vi "FP RT main.vi"() -> ()   [LabVIEW 2014]
uses:
  <vilib>/userdefined/High Color/IMAQdx.ctl
  <vilib>/myRIO/Instrument Drivers/Onboard IO/PWM/typedefs/PWM Reference.ctl
  <vilib>/myRIO/Common/Instrument Driver Framework/Utilities/typedefs/myRIO Generic Hardware Reference.ctl
  <vilib>/myRIO/Common/Instrument Driver Framework/Utilities/typedefs/Hardware Version Enum.ctl
  <vilib>/myRIO/Common/Instrument Driver Framework/Utilities/typedefs/myRIO v1.0 Reference.ctl
  <vilib>/myRIO/Common/Instrument Driver Framework/Utilities/typedefs/Generic FPGA Reference.ctl
  <vilib>/myRIO/Common/Instrument Driver Framework/myRIO v1.0/PWM/typedefs/PWM Channels Enum.ctl
  <vilib>/myRIO/Instrument Drivers/Onboard IO/PWM/typedefs/PWM Configuration.ctl
  <vilib>/userdefined/High Color/nirio_resource_hc.ctl
  <vilib>/myRIO/Instrument Drivers/Onboard IO/DIO/typedefs/DIO Reference.ctl
  <vilib>/myRIO/Common/Instrument Driver Framework/myRIO v1.0/DIO/typedefs/DIO Channels List.ctl
  <vilib>/myRIO/Common/Instrument Driver Framework/myRIO v1.0/DIO/typedefs/DIO Channels Enum.ctl
  <vilib>/myRIO/Instrument Drivers/Onboard IO/AI/typedefs/AI Reference.ctl
  <vilib>/myRIO/Common/Instrument Driver Framework/myRIO v1.0/AI/typedefs/AI Channels List.ctl
  <vilib>/myRIO/Common/Instrument Driver Framework/myRIO v1.0/AI/typedefs/AI Channels Enum.ctl
  <vilib>/myRIO/Common/Instrument Driver Framework/Utilities/typedefs/Analog Scaling Constants List.ctl
  <vilib>/myRIO/Common/Instrument Driver Framework/Utilities/typedefs/Analog Scaling Constants.ctl
  <vilib>/myRIO/Common/Instrument Driver Framework/myRIO v1.0/PWM/vis/myRIO v1.1 Open PWM.vi
  <vilib>/myRIO/Common/Instrument Driver Framework/myRIO v1.0/DIO/vis/myRIO v1.1 Open DIO.vi
  <vilib>/myRIO/Common/Instrument Driver Framework/myRIO v1.0/AI/vis/myRIO v1.1 Open AI.vi
  <vilib>/myRIO/Common/Instrument Driver Framework/Utilities/vis/Validate Channels.vi
  <vilib>/myRIO/Common/Instrument Driver Framework/myRIO v1.0/PWM/vis/myRIO v1.0 Reserve PWM.vi
  <vilib>/myRIO/Common/Instrument Driver Framework/myRIO v1.0/DIO/vis/myRIO v1.0 Reserve DIO.vi
  <vilib>/myRIO/Common/Instrument Driver Framework/myRIO v1.0/AI/vis/myRIO v1.0 Reserve AI.vi
  <vilib>/myRIO/Common/Instrument Driver Framework/myRIO v1.0/PWM/vis/myRIO v1.0 Close PWM.vi
  <vilib>/myRIO/Common/Instrument Driver Framework/myRIO v1.0/DIO/vis/myRIO v1.0 Close DIO.vi
  <vilib>/myRIO/Common/Instrument Driver Framework/myRIO v1.0/AI/vis/myRIO v1.0 Close AI.vi
  <vilib>/myRIO/Common/Instrument Driver Framework/myRIO v1.0/PWM/vis/myRIO v1.0 Build MUX Configuration PWM.vi
  <vilib>/myRIO/Common/Instrument Driver Framework/myRIO v1.0/Resource Manager/vis/myRIO v1.0 Reserve Channel List.vi
  <vilib>/myRIO/Common/Instrument Driver Framework/myRIO v1.0/DIO/vis/myRIO v1.0 Build MUX Configuration DIO.vi
  <vilib>/myRIO/Common/Instrument Driver Framework/myRIO v1.0/AI/vis/myRIO v1.0 Build MUX Configuration AI.vi
  <vilib>/myRIO/Common/Instrument Driver Framework/myRIO v1.0/PWM/vis/myRIO v1.0 Unreserve PWM.vi
  <vilib>/myRIO/Common/Instrument Driver Framework/myRIO v1.0/DIO/vis/myRIO v1.0 Unreserve DIO.vi
  <vilib>/myRIO/Common/Instrument Driver Framework/myRIO v1.0/AI/vis/myRIO v1.0 Unreserve AI.vi
  <vilib>/myRIO/Common/Instrument Driver Framework/myRIO v1.0/Resource Manager/vis/myRIO v1.0 Create Configuration List.vi
  <vilib>/myRIO/Common/Instrument Driver Framework/myRIO v1.0/Resource Manager/vis/myRIO v1.0 Reserve Channel.vi
  <vilib>/myRIO/Common/Instrument Driver Framework/myRIO v1.0/Resource Manager/vis/myRIO v1.0 Unreserve Channel.vi
  <vilib>/myRIO/Common/Instrument Driver Framework/myRIO v1.0/Resource Manager/vis/myRIO v1.0 Unreserve Channel List.vi
  <vilib>/myRIO/Common/Instrument Driver Framework/myRIO v1.0/Resource Manager/vis/myRIO v1.0 Build Mutex Name.vi
  <vilib>/Utility/VariantDataType/GetNumericInfo.vi
  <vilib>/Utility/error.llb/Error Cluster From Error Code.vi
  <vilib>/myRIO/Common/Instrument Driver Framework/myRIO v1.0/myRIO v1.1 Open.vi
  <vilib>/myRIO/Common/Instrument Driver Framework/myRIO v1.0/AI/vis/myRIO v1.0 Get Scaling Constants AI.vi
  <vilib>/myRIO/Common/Instrument Driver Framework/Utilities/vis/IO Manager.vi
  <vilib>/myRIO/Common/Instrument Driver Framework/Utilities/vis/Configuration Manager.vi
  <vilib>/myRIO/Common/Instrument Driver Framework/myRIO v1.0/myRIO v1.0 Close.vi
  <vilib>/myRIO/Common/Instrument Driver Framework/myRIO v1.0/Resource Manager/vis/myRIO v1.0 Configure IO.vi
  <vilib>/myRIO/Common/Instrument Driver Framework/myRIO v1.0/AI/vis/myRIO v1.0 Read AI.vi
  <vilib>/myRIO/Common/Instrument Driver Framework/myRIO v1.0/DIO/vis/myRIO v1.0 Write DIO.vi
  <vilib>/myRIO/Common/Instrument Driver Framework/myRIO v1.0/PWM/vis/myRIO v1.0 Write PWM.vi
  <vilib>/myRIO/Common/Instrument Driver Framework/myRIO v1.0/PWM/vis/myRIO v1.0 Shutdown PWM.vi
  <vilib>/myRIO/Common/Instrument Driver Framework/myRIO v1.0/DIO/vis/myRIO v1.0 Shutdown DIO.vi
  <vilib>/myRIO/Instrument Drivers/Onboard IO/AI/vis/myRIO AI Open.xnode
  <vilib>/myRIO/Instrument Drivers/Onboard IO/DIO/vis/myRIO DIO Open.xnode
  <vilib>/myRIO/Instrument Drivers/Onboard IO/PWM/vis/myRIO PWM Open.xnode
  <vilib>/vision/driver/NI_Vision_Acquisition_Software.lvlib
  <vilib>/myRIO/Instrument Drivers/Onboard IO/AI/AI.lvlib
  <vilib>/myRIO/Instrument Drivers/Onboard IO/DIO/DIO.lvlib
  <vilib>/myRIO/Instrument Drivers/Onboard IO/PWM/PWM.lvlib
panel:
  in  "Waypoint seed":T1={"Type"=enum."Start", "X"=250, "Y"=250, "Speed"=0, "Behaviors"=enum."Open Water Transit"}
  in  "spyder":cluster{"magnitude":dbl, "phase":dbl}[](array[cluster]) {"phase" format="%0.2f"; "magnitude" format="%0.2f"}
  in  "Tab Control":T2(tab)
  out "GLED":bool
  out "BLED":bool
  out "RLED":bool
  out "BW Image":T3(plugin-control)
  in  "stop":bool
  out "Midbrain?":bool
  out "Rudder":dbl(knob) min=-45.0 max=45.0 step=1.0 scale=-45.0..45.0
  out "Speed":dbl(knob) min=-9.0 max=9.0 step=1.0 scale=-50.0..50.0
  out "Hindbrain?":bool
  out "Forebrain?":bool
  out "Battery Dead?":bool
  out "Complete?":bool=TRUE
  out "Arbiter Graph":cluster{dbl, dbl, dbl[]}(graph)
  in  "Session In":T4="cam0"
  out "Color Image":T3(plugin-control)
  out "Nb Circles":i32
  out "UDP Time Out?":bool
  in  "Tug letter":string="T"
  in  "Run?":bool
  in  "MSpeed":dbl(slide) scale=-50.0..50.0 scale format="%#.1g"
  in  "MHeading":dbl(slide) scale=-45.0..45.0 scale format="%_1f"
  in  "Manual?":bool
  out "Boat Status":T5={"GPS"={"X pos"=0, "Y pos"=0, "Heading"=0.0}, "IR Sensors"=[{"Name"="Bow", "Angle"=0.0, "Distance"=0.0}], "MOT BAT"=7.2, "RIO BAT"=7.2}
  out "GPS?":bool
  out "Camera Data":T6
  out "TA GPS":cluster{"X pos":i32, "Y pos":i32, "Heading":dbl}
  in  "TA Tug Letter":string="L"
  out "TAGPS?":bool
  out "Act Com":T7
  out "Forebrain ACT":dbl[](array[numeric])
  out "IR Sensors":T8(array[cluster])
  out "GPS":cluster{"X pos":i32, "Y pos":i32, "Heading":dbl}
  out "RED LED":bool
  out "GREEN LED":bool
  out "BLUE LED":bool
  in  "MDF":T9(array[cluster])=[{"Type"=enum."Start", "X"=250, "Y"=250, "Speed"=0, "Behaviors"=enum."Open Water Transit"}, {"Type"=enum."Waypoint", "X"=400, "Y"=100, "Speed"=20, "Behaviors"=enum."P-Wall Follow"}, {"Type"=enum."Waypoint", "X"=250, "Y"=250, "Speed"=20, "Behaviors"=enum."Open Water Transit"}, {"Type"=enum."Waypoint", "X"=250, "Y"=400, "Speed"=20, "Behaviors"=enum."Open Water Transit"}, {"Type"=enum."Waypoint", "X"=100, "Y"=400, "Speed"=20, "Behaviors"=enum."Open Water Transit"}, {"Type"=enum."End", "X"=250, "Y"=250, "Speed"=0, "Behaviors"=enum."Open Water Transit"}]
  out "GPS Initial":cluster{"X pos":i32, "Y pos":i32, "Heading":dbl}
  out "In chase mode?":bool
  out "Polar Plot":picture
  out "Invalid Pos?":bool
  out "error out":errorcluster
  out "Forebrain Comd":T10
  out "Debug IR \nRaw \nReadings":T8(array[cluster])
  out "Boat Speed":dbl format="%#_15g"
  in  "BOATPOS":T11
  in  "Boxcars":T12
  out "Chase MDF":T9(array[cluster])
  out "MDF INDEX CHASE":i32
  out "Docking MDF":T9(array[cluster])
  out "MDF INDEX DOCKING":i32
  out "MDF Active":T9(array[cluster])
  out "MDF INDEX":i32
  # "To start the Tug, press the \">\" key in the tool bar.\n\nPress the Run? control to start the Mission.\n\nWhen complete the Complete? indicator will light.\n\nIf the Run? is not pressed again, the mission will start again.\n\nAlways press the STOP button to end the operation!!!!!!!!!!!!!"
  # "Press the Manual? button to control\nthe Tug from the sliders"
  # "Stuck indicates that\nthe boat is not moving."
  # "Enter the Letter\nof  your Tug"
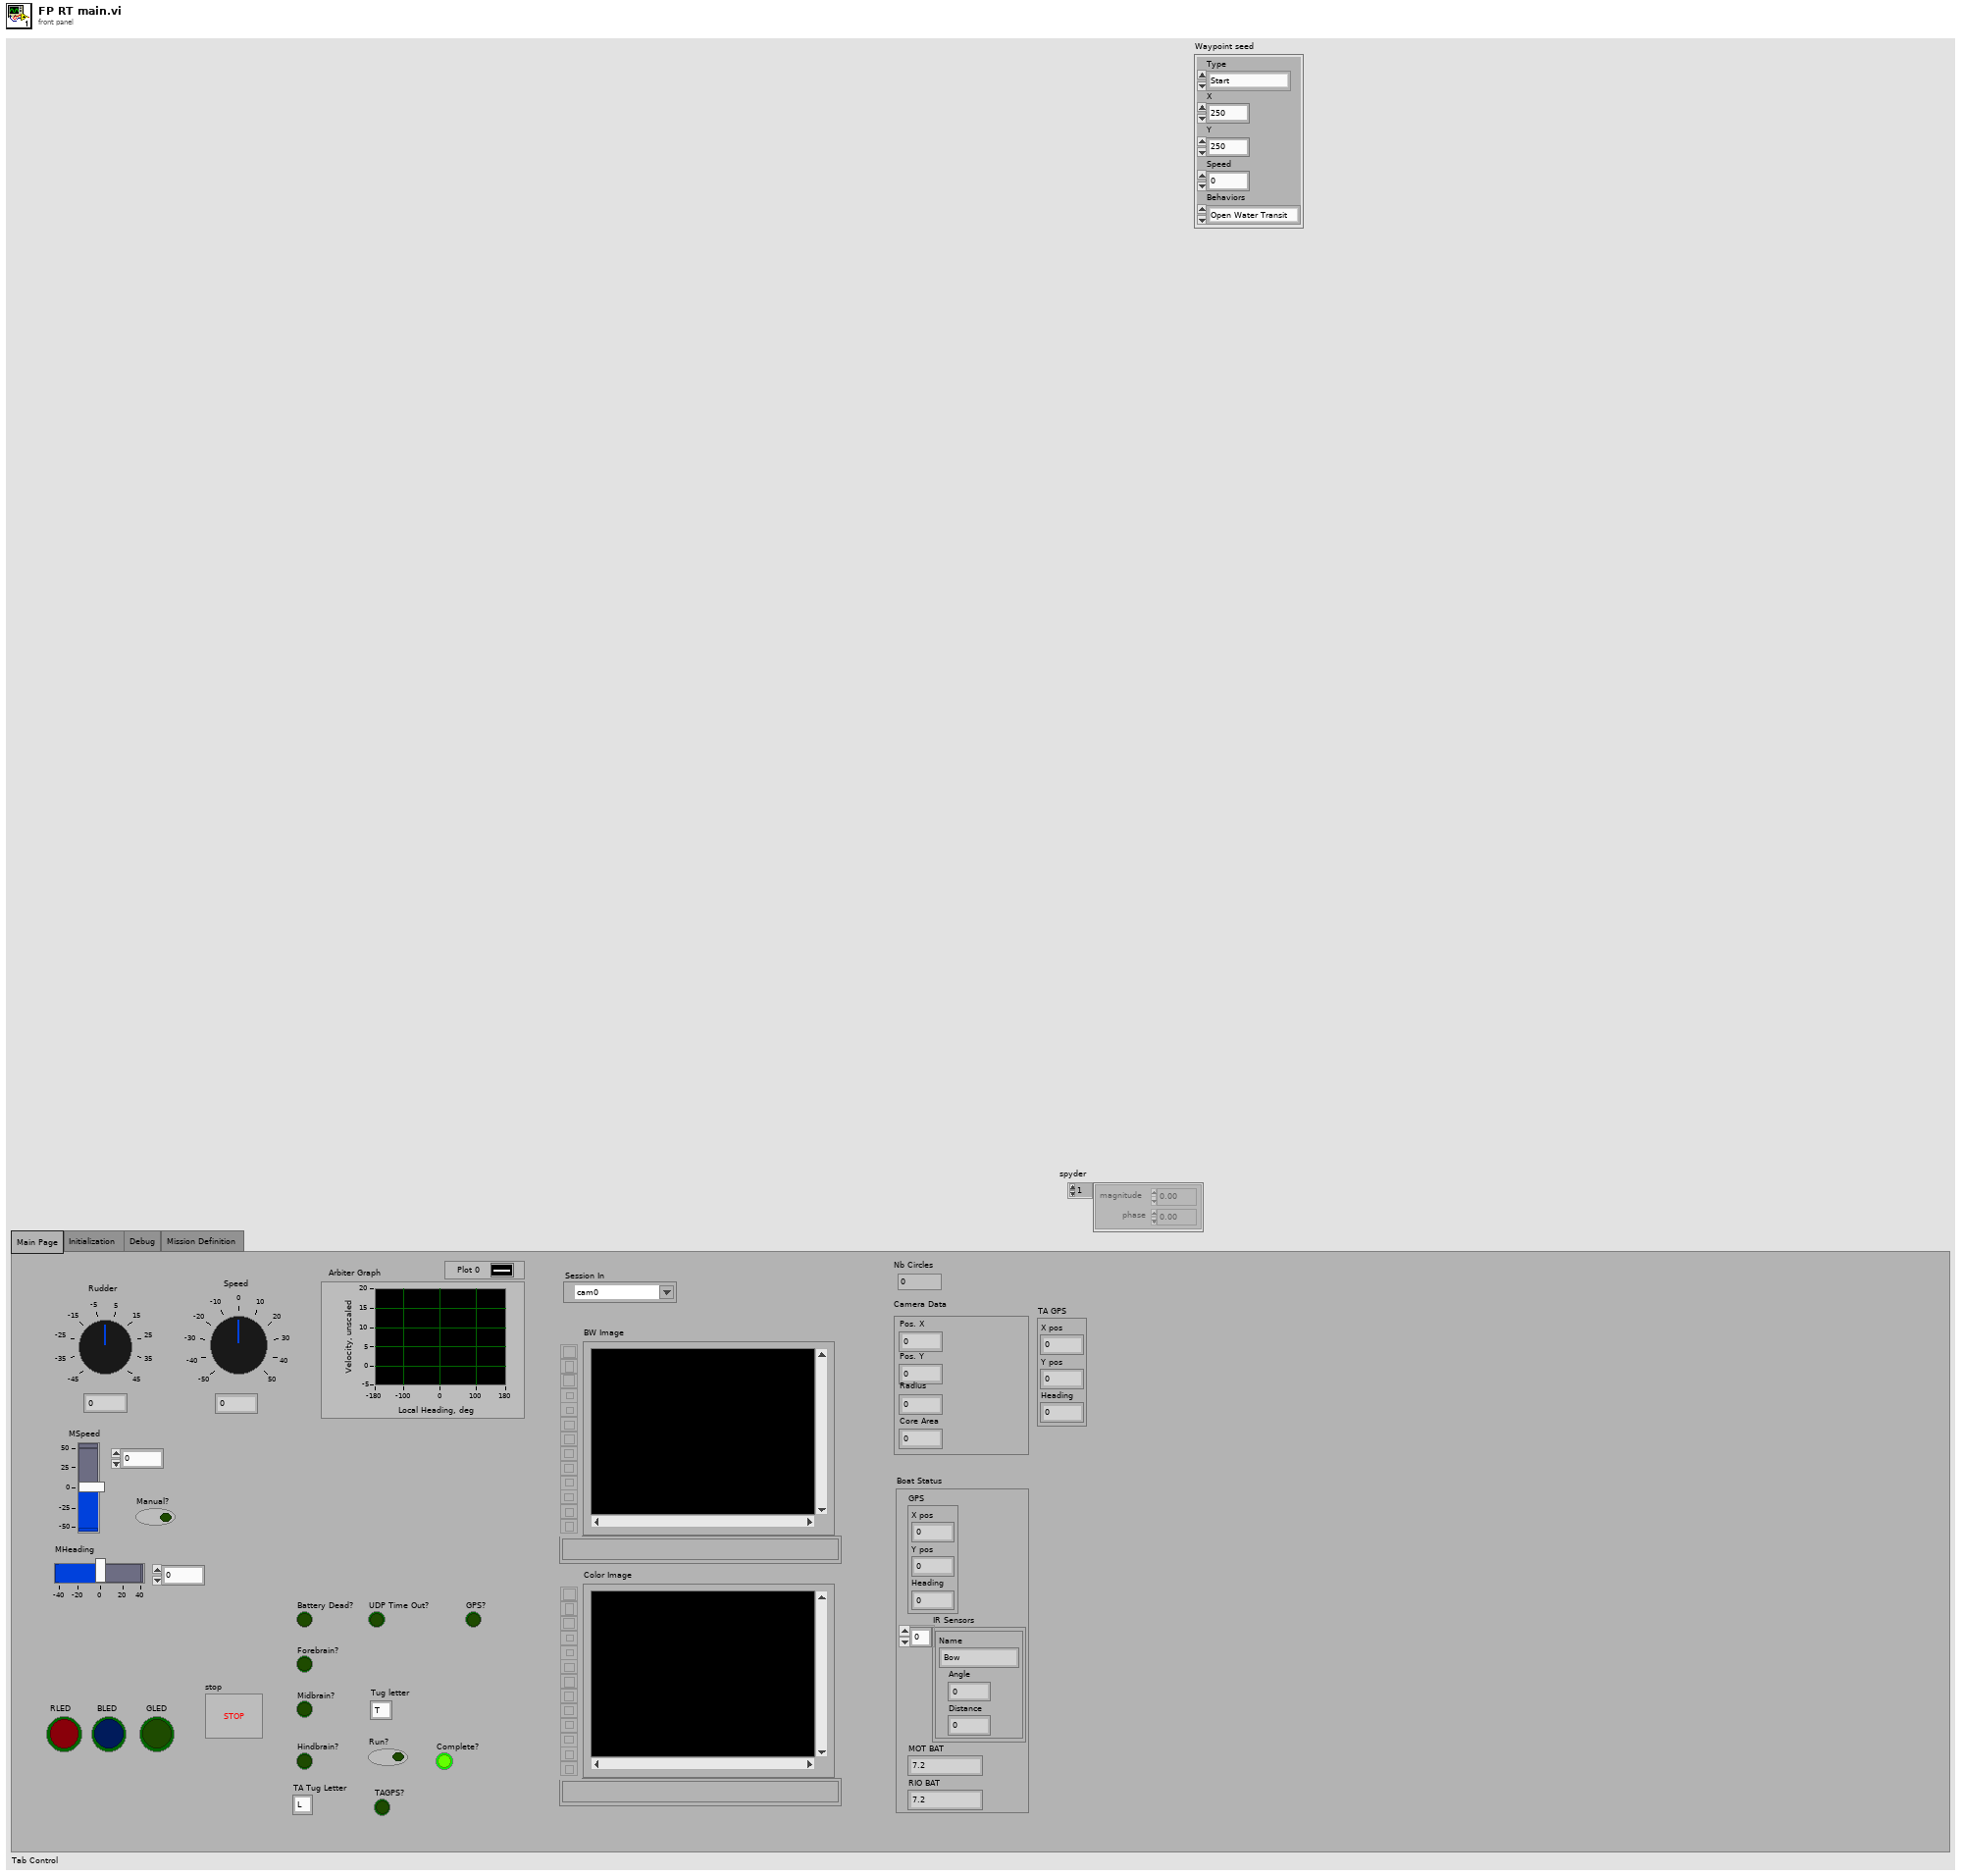
[diagram p1: front panel]
types:
  T1 = cluster{"Type":enum16{"Start", "Waypoint", "End"}, "X":i32, "Y":i32, "Speed":i32, "Behaviors":enum16{"Open Water Transit", "P-Wall Follow", "S-Wall Follow", "Dock", "Chase"}}
  T2 = enum32{"Main Page", "Initialization", "Debug", "Mission Definition"}
  T3 = typedef "IMAQ Image.ctl" = refnum<image>
  T4 = typedef "IMAQdx.ctl" = refnum<k21>
  T5 = cluster{"GPS":cluster{"X pos":i32, "Y pos":i32, "Heading":dbl}, "IR Sensors":cluster{"Name":string, "Angle":dbl, "Distance":dbl}[], "MOT BAT":dbl, "RIO BAT":dbl}
  T6 = cluster{"Pos. X":i32, "Pos. Y":i32, "Radius":i32, "Core Area":i32}
  T7 = cluster{"Desired Local\nHeading":dbl, "Desired\nSpeed":dbl}
  T8 = cluster{"Name":string, "Angle":dbl, "Distance":dbl}[]
  T9 = cluster{"Type":enum16{"Start", "Waypoint", "End"}, "X":i32, "Y":i32, "Speed":i32, "Behaviors":enum16{"Open Water Transit", "P-Wall Follow", "S-Wall Follow", "Dock", "Chase"}}[]
  T10 = cluster{"Behaviors":enum16{"Open Water Transit", "P-Wall Follow", "S-Wall Follow", "Dock", "Chase"}, "Behavior\nVelocity":dbl}
  T11 = cluster{"Old X Position":i32, "Old Y Position":i32}
  T12 = cluster{"IR Sensor Boxcars":dbl[][], "Boat Speed  Boxcars":dbl[]}
  T13 = cluster{"Type":enum16{"Start", "Waypoint", "End"}, "X":i32, "Y":i32, "Speed":i32, "Behaviors":enum16{"Open Water Transit", "P-Wall Follow", "S-Wall Follow", "Dock"}}[]
  T14 = typedef "nirio_resource_hc.ctl" = tag
  T15 = typedef "Hardware Version Enum.ctl" = enum16{"Unknown", "myRIO-1900", "myRIO-1950"}
  T16 = typedef "Image Type" = u32
  T17 = enum16{"Open Water Transit", "P-Wall Follow", "S-Wall Follow", "Dock", "Chase"}
  T18 = typedef "PWM.lvlib/PWM Reference.ctl" = cluster{"myRIO Reference":T19, "PWM Channels Enum":T22, "PWM Configuration":T23}
  T19 = typedef "myRIO Generic Hardware Reference.ctl" = cluster{"myRIO Model":T15, "myRIO Hardware Reference":T20}
  T20 = typedef "myRIO v1.0 Reference.ctl" = cluster{"Generic FPGA Reference":T21, "Allow multiple opens":bool}
  T21 = typedef "Generic FPGA Reference.ctl" = refnum<k20>
  T22 = typedef "PWM Channels Enum.ctl" = enum16{"Not Connected", "C/PWM0", "C/PWM1", "A/PWM0", "A/PWM1", "A/PWM2", "B/PWM0", "B/PWM1", "B/PWM2"}
  T23 = typedef "PWM.lvlib/PWM Configuration.ctl" = cluster{"Frequency":dbl, "Duty Cycle":dbl}
  T24 = typedef "DIO.lvlib/DIO Reference.ctl" = cluster{"myRIO Reference":T19, "DIO Channels List":T25}
  T25 = typedef "DIO Channels List.ctl" = T26[]
  T26 = typedef "DIO Channels Enum.ctl" = enum16{"Not Connected", "C/DIO0", "C/DIO1", "C/DIO2", "C/DIO3", "C/DIO4", "C/DIO5", "C/DIO6", "C/DIO7", "A/DIO0", "A/DIO1", "A/DIO2", "A/DIO3", "A/DIO4", "A/DIO5", "A/DIO6", "A/DIO7", "A/DIO8", "A/DIO9", "A/DIO10", "A/DIO11", "A/DIO12", "A/DIO13", "A/DIO14", "A/DIO15", "B/DIO0", "B/DIO1", "B/DIO2", "B/DIO3", "B/DIO4", "B/DIO5", "B/DIO6", "B/DIO7", "B/DIO8", "B/DIO9", "B/DIO10", "B/DIO11", "B/DIO12", "B/DIO13", "B/DIO14", "B/DIO15", "LED0", "LED1", "LED2", "LED3", "Button0"}
  T27 = typedef "AI.lvlib/AI Reference.ctl" = cluster{"myRIO Reference":T19, "AI Channels List":T28, "AI Scaling Constants List":T30}
  T28 = typedef "AI Channels List.ctl" = T29[]
  T29 = typedef "AI Channels Enum.ctl" = enum16{"Not Connected", "AudioIn/Left", "AudioIn/Right", "C/AI0", "C/AI1", "A/AI0", "A/AI1", "A/AI2", "A/AI3", "B/AI0", "B/AI1", "B/AI2", "B/AI3"}
  T30 = typedef "Analog Scaling Constants List.ctl" = T31[]
  T31 = typedef "Analog Scaling Constants.ctl" = cluster{"LSB Weight (Volts)":dbl, "Offset (Volts)":dbl, "Signed?":bool}
  T32 = cluster{"New X Position":i32, "New Y Position":i32}
  T33 = cluster{"regular expression":string, i32, i32, i32}
  T34 = cluster{"maximum":dbl, "minimum":dbl, "clip to min":bool, "log?(F)":bool, "grid color":u32, "plot color":u32, "fmt and prec":cluster{"format":enum8{"Decimal", "Scientific", "Engineering", "Binary", "Octal", "Hex"}, "precision":u8}, "visible section":u16}
  T35 = typedef "LVBoundsTypeDef.ctl" = cluster{"Width":u32, "Height":u32}
  T36 = cluster{"Obs Avoid Array":dbl[], "P-Wall Array":dbl[], "S-Wall Array":dbl[], "Docking Array":dbl[]}
  T37 = cluster{"Behaviors":enum16{"Open Water Transit", "P-Wall Follow", "S-Wall Follow", "Dock", "Chase"}, dbl}
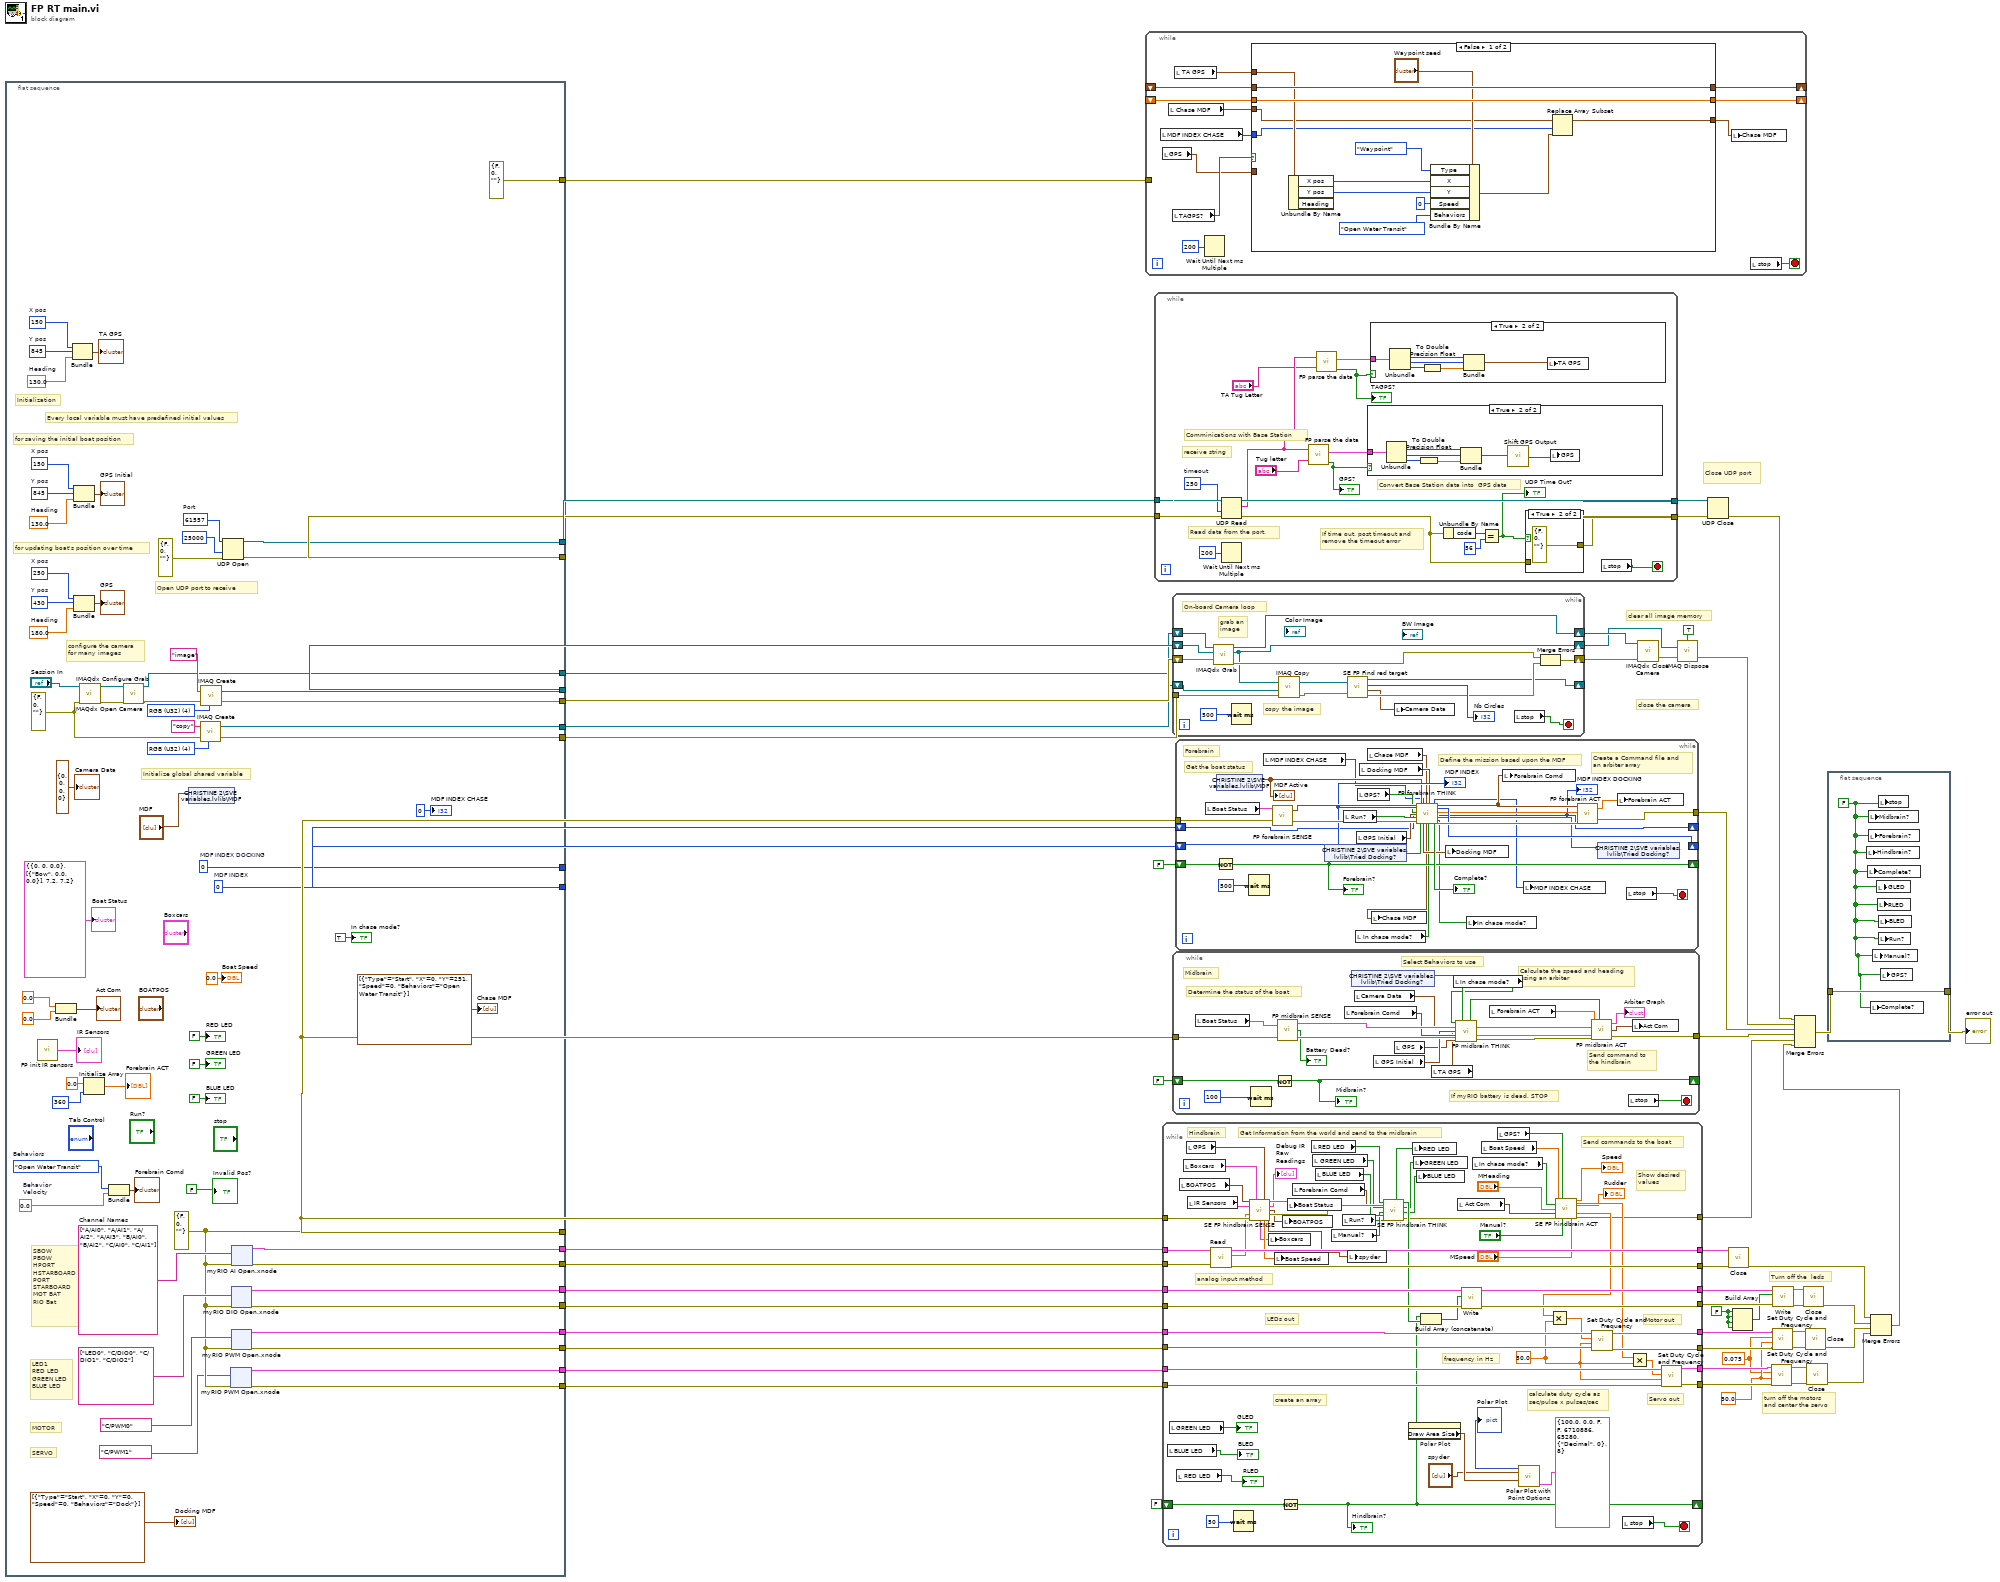
[diagram p0: block diagram]
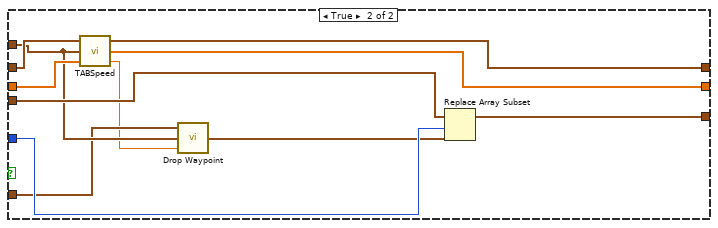
[diagram p2: hidden frame]
diagram:
  w9 = 0.075
  w8 = FALSE
  w10 = 50.0
  # "Turn off the  leds"
  # "turn off the motors\nand center the servo"
  # "Close UDP port"
  # "clear all image memory"
  # "close the camera"
  n1 = flat-sequence {
    tunnel: [w86] -> w56
    tunnel: [w120] -> w53
    tunnel: [w112] -> w52
    tunnel: [w111] -> w51
    tunnel: [w110] -> w50
    tunnel: [w106] -> w43
    tunnel: [w105] -> w44
    tunnel: [w101] -> w3
    tunnel: [w100] -> w2
    tunnel: [w94] -> w38
    tunnel: [w93] -> w37
    tunnel: [w91] -> w33
    tunnel: [w90] -> w34
    tunnel: [w88] -> w32
    tunnel: [w87] -> w31
    tunnel: [w84] -> w30
    tunnel: [w83] -> w29
    tunnel: [w69] -> w4
    tunnel: [errorcluster {"status"=FALSE, "code"=0, "source"=""} ("error in")] -> w1
    frame #0 {
      w63 = 845  # Y pos
      w62 = 150  # X pos
      w61 = 130.0  # Heading
      w69 = 0  # MDF INDEX DOCKING
      w72 = 845  # Y pos
      w73 = 150  # X pos
      w74 = 130.0  # Heading
      w95 = tag[] ["A/AI0", "A/AI1", "A/AI2", "A/AI3", "B/AI0", "B/AI2", "C/AI0", "C/AI1"]  # Channel Names
      w97 = 430  # Y pos
      w98 = 250  # X pos
      w99 = 180.0  # Heading
      w104 = u16 61557  # Port
      w109 = T16 4 items=["Grayscale (U8)", "Grayscale (I16)", "Grayscale (SGL)", "Complex (CSG)", "RGB (U32)", "HSL (U32)", "RGB (U64)", "Grayscale (U16)"] ("Image Type")
      w107 = errorcluster {"status"=FALSE, "code"=0, "source"=""} ("error in")
      w117 = T16 4 items=["Grayscale (U8)", "Grayscale (I16)", "Grayscale (SGL)", "Complex (CSG)", "RGB (U32)", "HSL (U32)", "RGB (U64)", "Grayscale (U16)"] ("Image Type")
      w86 = errorcluster {"status"=FALSE, "code"=0, "source"=""} ("error out")
      w120 = 0  # MDF INDEX
      w124 = 0.0  # Behavior Velocity
      w119 = T17."Open Water Transit"  # Behaviors
      # "for saving the initial boat position"
      # "Initialize global shared variable"
      # "LED1\nRED LED\nGREEN LED\nBLUE LED"
      # "SERVO"
      # "MOTOR"
      # "SBOW\nPBOW\nHPORT\nHSTARBOARD\nPORT\nSTARBOARD\nMOT BAT\nRIO Bat"
      # "for updating boat's position over time"
      # "Open UDP port to receive"
      # "configure the camera\nfor many images"
      # "Every local variable must have predefined initial values"
      # "Initialization"
      n2 = call "FP init IR sensors.vi"() -> ("IR Sensors"=→"IR Sensors":T8)  [unwired: 1 in]
      n3 = Bundle(0.0, 0.0) -> (→"Act Com":cluster{dbl, dbl})  [unwired: 1 in]
      n4 = Bundle("X pos"=w62, "Y pos"=w63, "Heading"=w61) -> (→"TA GPS":cluster{"X pos":i32, "Y pos":i32, "Heading":dbl})  [unwired: 1 in]
      n5 = Bundle("X pos"=w73, "Y pos"=w72, "Heading"=w74) -> (→"GPS Initial":cluster{"X pos":i32, "Y pos":i32, "Heading":dbl})  [unwired: 1 in]
      n6 = Bundle("X pos"=w98, "Y pos"=w97, "Heading"=w99) -> (→"GPS":cluster{"X pos":i32, "Y pos":i32, "Heading":dbl})  [unwired: 1 in]
      n7 = call <vilib>:"IMAQdx Open Camera.vi"("error in"=w107, "Session In"="Session In") -> ("error out"=w114:errorcluster, "Session Out"=w113:T4)  [unwired: 1 in, 7 out]
      n8 = Initialize Array(0.0 ("element"), 360 ("dimension size")) -> (→"Forebrain ACT":dbl[])
      n9 = Bundle("Behaviors"=w119, "Behavior\nVelocity"=w124) -> (→"Forebrain Comd":T10)  [unwired: 1 in]
      n10 = call <vilib>:"IMAQdx Configure Grab.vi"("error in"=w114, "Session In"=w113) -> ("error out"=w118:errorcluster, "Session Out"=w110:T4)  [unwired: 8 out]
      n11 = shared-variable "CHRISTINE 2\\SVE variables.lvlib\\MDF"("MDF") -> ()  [unwired: 1 in, 1 out]
      n12 = call "IMAQ Create"("Image Name"="copy", "Image Type"=w109, "error in (no error)"=w107) -> ("New Image"=w105:T3, "error out"=w106:errorcluster)  [unwired: 2 in]
      n13 = call "IMAQ Create"("Image Name"="image", "Image Type"=w117, "error in (no error)"=w118) -> ("New Image"=w111:T3, "error out"=w112:errorcluster)  [unwired: 1 in, 1 out]
      n14 = UDP Open(8:errorcluster {"status"=FALSE, "code"=0, "source"=""} ("error in"), 9:25000 ("timeout ms (25000)"), 11:w104) -> (port=w101:refnum<k16>, 0:w100:errorcluster)  [unwired: 2 in, 1 out]
      n15 = xnode "myRIO PWM Open.xnode"("error in (no error)"=w86, "Channel Name"=tag "C/PWM1") -> ("error out"=w84:errorcluster, "PWM Ref Out"=w83:T18)  [unwired: 1 in]
      n16 = xnode "myRIO DIO Open.xnode"("error in (no error)"=w86, "Channel Names"=tag[] ["LED0", "C/DIO0", "C/DIO1", "C/DIO2"]) -> ("error out"=w91:errorcluster, "DIO Ref Out"=w90:T24)  [unwired: 1 in]
      n17 = xnode "myRIO PWM Open.xnode"("error in (no error)"=w86, "Channel Name"=tag "C/PWM0") -> ("error out"=w88:errorcluster, "PWM Ref Out"=w87:T18)  [unwired: 1 in]
      n18 = xnode "myRIO AI Open.xnode"("error in (no error)"=w86, "Channel Names"=w95) -> ("error out"=w94:errorcluster, "AI Ref Out"=w93:T27)  [unwired: 1 in]
      "Invalid Pos?" <- FALSE
      "RED LED" <- FALSE ("RED LED")
      "GREEN LED" <- FALSE ("GREEN LED")
      "BLUE LED" <- FALSE ("WHITE LED")
      "Boat Status" <- T5 {"GPS"={"X pos"=0, "Y pos"=0, "Heading"=0.0}, "IR Sensors"=[{"Name"="Bow", "Angle"=0.0, "Distance"=0.0}], "MOT BAT"=7.2, "RIO BAT"=7.2} ("Boat Status 2")
      "Boat Speed" <- 0.0 ("Boat Speed")
      "Docking MDF" <- T13 [{"Type"=enum."Start", "X"=0, "Y"=0, "Speed"=0, "Behaviors"=enum."Dock"}] ("Docking MDF")
      "Camera Data" <- T6 {"Pos. X"=0, "Pos. Y"=0, "Radius"=0, "Core Area"=0} ("Camera Data")
      "In chase mode?" <- TRUE ("In chase mode?")
      "Chase MDF" <- T9 [{"Type"=enum."Start", "X"=0, "Y"=251, "Speed"=0, "Behaviors"=enum."Open Water Transit"}] ("Chase MDF")
      "MDF INDEX CHASE" <- 0 ("MDF INDEX CHASE")
    }
  }
  n19 = while {
    tunnel: w1 -> [_]
    shift-right: [w201] -> _
    shift-left: _ -> [w202]
    shift-right: [w199] -> _
    shift-left: _ -> [w200]
    stop <- w197 stop-if-true
    n20 = local read "MDF INDEX CHASE"() -> (w204:i32)
    n21 = local read "GPS"() -> (w195:cluster{"X pos":i32, "Y pos":i32, "Heading":dbl})
    n22 = local read "Chase MDF"() -> (w205:T9)
    n23 = local read "TAGPS?"() -> (w196:bool)
    n24 = local read "TA GPS"() -> (w203:cluster{"X pos":i32, "Y pos":i32, "Heading":dbl})
    n25 = Wait Until Next ms Multiple(millisecond multiple=u32 200) -> ()  [unwired: 1 out]
    n26 = case shown="False" w196 {
      tunnel: w205 -> [w210 w225]
      tunnel: w204 -> [w207 w227]
      tunnel: w203 -> [w213 w224]
      tunnel: w202 -> [w219 w230]
      tunnel: [w219 w229] -> w201
      tunnel: w200 -> [w218 w228]
      tunnel: [w218 w223] -> w199
      tunnel: [w209 w226] -> w198
      tunnel: w195 -> [_ w222]
      frame False {
        n27 = Unbundle By Name(w213) -> ("X pos"=w212:i32, "Y pos"=w211:i32)  [unwired: 1 out]
        n28 = Bundle By Name(cluster="Waypoint seed", "Type"=enum16{"Start", "Waypoint", "End"}."Waypoint", "X"=w212, "Y"=w211, "Speed"=0, "Behaviors"=T17."Open Water Transit") -> (w208:T1)
        n29 = Replace Array Subset(array=w210, new element=w208, index=w207) -> (w209:T9)
      }
      frame True {
        n30 = call "TABSpeed.vi"("Boxcar Average"=w228, "Current Position"=w224, "Old Position"=w230) -> ("New Speed of Boat\nin Pixels/Sec"=w221:dbl, "Boxcar Average Out"=w223:dbl[], "New Position"=w229:T32)
        n31 = call "Drop Waypoint.vi"("TA Speed"=w221, "TA GPS"=w224, "Our GPS"=w222) -> ("Output Waypoint"=w220:T1)
        n32 = Replace Array Subset(array=w225, new element=w220, index=w227) -> (w226:T9)
      }
    }
    n33 = local write "Chase MDF"(w198) -> ()
    n34 = local read "stop"() -> (w197:bool)
  }
  n35 = while {
    tunnel: w2 -> [w248]
    tunnel: w3 -> [w247]
    tunnel: [w246] -> w41
    tunnel: [w241] -> w40
    stop <- w238 stop-if-true
    w240 = 250  # timeout
    # "Convert Base Station data into  GPS data"
    # "Comminications with Base Station"
    # "receive string"
    # "If time out, post timeout and\nremove the timeout error"
    # "Read data from the port."
    n36 = UDP Read(connection ID=w247, timeout ms (25000)=w240, 8:w248) -> (data out=w235:string, error out=w242:errorcluster, 3:w246:refnum<k16>)  [unwired: 1 in, 2 out]
    n37 = Wait Until Next ms Multiple(millisecond multiple=u32 200) -> ()  [unwired: 1 out]
    n38 = call "FP parse the data.vi"("Nav String"=w235, "Tug"="Tug letter") -> ("Tug Location"=w236:T33, "Valid?"=w232:bool)  [unwired: 2 out]
    "GPS?" <- w232
    n39 = call "FP parse the data.vi"("Nav String"=w235, "Tug"="TA Tug Letter") -> ("Tug Location"=w233:T33, "Valid?"=w231:bool)  [unwired: 2 out]
    "TAGPS?" <- w231
    n40 = case shown="True" w232 {
      tunnel: w236 -> [_ w261]
      frame False {
      }
      frame True {
        n41 = Unbundle(w261) -> (w260:i32, w259:i32, w257:i32)  [unwired: 1 out]
        n42 = To Double Precision Float(number=w257) -> (double precision float=w258:dbl)
        n43 = Bundle(w260, w259, w258) -> (w256:cluster{i32, i32, dbl})  [unwired: 1 in]
        n44 = call "Shift GPS Output.vi"("GPS Input"=w256) -> ("GPS Output"=w255:cluster{"X pos":i32, "Y pos":i32, "Heading":dbl})
        n45 = local write "GPS"(w255) -> ()
      }
    }
    n46 = case shown="True" w231 {
      tunnel: w233 -> [_ w254]
      frame False {
      }
      frame True {
        n47 = Unbundle(w254) -> (w253:i32, w252:i32, w250:i32)  [unwired: 1 out]
        n48 = To Double Precision Float(number=w250) -> (double precision float=w251:dbl)
        n49 = Bundle(w253, w252, w251) -> (w249:cluster{i32, i32, dbl})  [unwired: 1 in]
        n50 = local write "TA GPS"(w249) -> ()
      }
    }
    n51 = Unbundle By Name(w242) -> ("code"=w245:i32)
    n52 = Equal?(x=w245, y=56) -> (x = y?=w243:bool)
    "UDP Time Out?" <- w243
    n53 = case shown="True" w243 {
      tunnel: [w262 errorcluster {"status"=FALSE, "code"=0, "source"=""} ("error out")] -> w241
      tunnel: w242 -> [w262 _]
      frame False {
      }
      frame True {
      }
    }
    n54 = local read "stop"() -> (w238:bool)
  }
  n55 = while {
    tunnel: w56 -> [w328]
    shift-right: [w292] -> _
    shift-left: FALSE -> [w317]
    tunnel: w38 -> [w325]
    tunnel: w37 -> [w324]
    tunnel: [w323] -> w36
    tunnel: [w322] -> w35
    tunnel: w34 -> [w320]
    tunnel: w33 -> [w321]
    tunnel: [w319] -> w15
    tunnel: [w318] -> w12
    tunnel: w32 -> [w315]
    tunnel: w31 -> [w316]
    tunnel: [w314] -> w24
    tunnel: [w313] -> w21
    tunnel: w30 -> [w312]
    tunnel: [w311] -> w28
    tunnel: w29 -> [w310]
    tunnel: [w309] -> w26
    tunnel: [w276] -> w5
    stop <- w330 stop-if-true
    w304 = 50.0
    # "create an array"
    # "frequency in Hz"
    # "calculate duty cycle as\nsec/pulse x pulses/sec"
    # "Show desired\nvalues"
    # "Motor out"
    # "Servo out"
    # "LEDs out"
    # "analog input method"
    # "Send commands to the boat"
    # "Get Information from the world and send to the midbrain"
    # "Hindbrain"
    n56 = local read "BLUE LED"() -> (→"BLED":bool)
    n57 = local read "GREEN LED"() -> (→"GLED":bool)
    n58 = local read "RED LED"() -> (→"RLED":bool)
    n59 = local read "BOATPOS"() -> (w273:T11)
    n60 = local read "Boxcars"() -> (w271:T12)
    n61 = local read "GPS"() -> (w326:cluster{"X pos":i32, "Y pos":i32, "Heading":dbl})
    n62 = local read "IR Sensors"() -> (w290:T8)
    n63 = call <vilib>:"Read.vi"("error in (no error)"=w325, "AI Ref In"=w324) -> ("error out"=w323:errorcluster, "Values"=w308:dbl[], "AI Ref Out"=w322:T27)  [unwired: 7 in]
    n64 = Wait (ms)(milliseconds to wait=u32 50) -> ()  [unwired: 1 out]
    n65 = call "SE FP hindbrain SENSE.vi"("Old Position"=w273, "Boxcars In"=w271, "GPS"=w326, "IR Sensors"=w290, "Analog Input Values"=w308, "error in"=w328) -> ("Boat Status"=w291:T5, "IR Sensors 2"=→"Debug IR \nRaw \nReadings":T8, "New Position"=w272:T32, "error out"=w327:errorcluster, "Boxcars Out"=w270:T12, "New Speed of Boat\nin Pixels/Sec"=w279:dbl, "spyder"=w265:cluster{"magnitude":dbl, "phase":dbl}[])  [unwired: 3 in]
    n66 = local write "Boxcars"(w270) -> ()
    n67 = local write "Boat Speed"(w279) -> ()
    n68 = Not(x=w317) -> (.not. x?=w292:bool)
    "Hindbrain?" <- w292
    n69 = local write "BOATPOS"(w272) -> ()
    n70 = local write "Boat Status"(w291) -> ()
    n71 = local read "Forebrain Comd"() -> (w289:T10)
    n72 = local read "RED LED"() -> (w295:bool)
    n73 = local read "GREEN LED"() -> (w294:bool)
    n74 = local read "BLUE LED"() -> (w293:bool)
    n75 = local read "Manual?"() -> (w285:bool)
    n76 = local read "Run?"() -> (w280:bool)
    n77 = local write "spyder"(w265) -> ()
    n78 = call "SE FP hindbrain THINK.vi"("error in"=w327, "BLUE LED"=w293, "Forebrain Comd"=w289, "RUN?"=w280, "MANUAL"=w285, "GREEN LED"=w294, "RED LED"=w295) -> ("error out"=w277:errorcluster, "BLUE LED OUT"=w286:bool, "GREEN LED OUT"=w287:bool, "LED array"=w297:bool[], "RED LED OUT"=w288:bool)
    n79 = property on="Polar Plot" class="Pict"() -> ("Draw Area Size"=w268:T35)  [unwired: 2 in, 2 out]
    n80 = local write "RED LED"(w288) -> ()
    n81 = local write "GREEN LED"(w287) -> ()
    n82 = local write "BLUE LED"(w286) -> ()
    n83 = Build Array (concatenate)(w292, w297) -> (w296:bool[])
    n84 = local read "Act Com"() -> (w301:T7)
    n85 = call <vilib>:"Write.vi"("error in (no error)"=w321, "Values"=w296, "DIO Ref In"=w320) -> ("error out"=w319:errorcluster, "DIO Ref Out"=w318:T24)  [unwired: 6 in]
    n86 = local read "In chase mode?"() -> (w264:bool)
    n87 = local read "Boat Speed"() -> (w278:dbl)
    n88 = local read "GPS?"() -> (w275:bool)
    n89 = call <vilib>:"Polar Plot with Point Options.vi"("data array [mag, phase (deg)]"="spyder", "dimensions (w,h)"=w268, "polar attributes"=T34 {"maximum"=100.0, "minimum"=0.0, "clip to min"=FALSE, "log?(F)"=FALSE, "grid color"=6710886, "plot color"=65280, "fmt and prec"={"format"=enum."Decimal", "precision"=0}, "visible section"=8}) -> ("new picture"=→"Polar Plot":picture)  [unwired: 12 in]
    n90 = call "SE FP hindbrain ACT.vi"("Current Boat Speed"=w278, "GPS?"=w275, "Chase Mode?"=w264, "MHeading"="MHeading", "Act Com"=w301, "error in"=w277, "Manual?"="Manual?", "MSpeed"="MSpeed") -> ("Rudder"=w305:dbl, "Desired\nSpeed"=→"Speed":dbl, "Desired \nRudder"=→"Rudder":dbl, "Speed"=w307:dbl, "error out"=w276:errorcluster)  [unwired: 3 in]
    n91 = Multiply(x=w307, y=w304) -> (x*y=w306:dbl)
    n92 = call <vilib>:"Set Duty Cycle and Frequency.vi"("error in (no error)"=w315, "Frequency [Hz]"=w304, "Duty Cycle"=w306, "PWM Ref In"=w316) -> ("error out"=w314:errorcluster, "PWM Ref Out"=w313:T18)  [unwired: 5 in]
    n93 = local read "stop"() -> (w330:bool)
    n94 = Multiply(x=w305, y=w304) -> (x*y=w303:dbl)
    n95 = call <vilib>:"Set Duty Cycle and Frequency.vi"("error in (no error)"=w312, "Frequency [Hz]"=w304, "Duty Cycle"=w303, "PWM Ref In"=w310) -> ("error out"=w311:errorcluster, "PWM Ref Out"=w309:T18)  [unwired: 5 in]
  }
  n96 = while {
    shift-right: [w334] -> w48
    shift-left: w52 -> [w346]
    shift-right: [w333] -> w46
    shift-left: w51 -> [w345]
    shift-right: [w338] -> w47
    shift-left: w50 -> [w344]
    tunnel: w43 -> [w342]
    shift-right: [w332] -> _
    shift-left: w44 -> [w341]
    stop <- w347 stop-if-true
    # "grab an\nimage"
    # "copy the image"
    # "On-board Camera loop"
    n97 = call <vilib>:"IMAQdx Grab.vi"("error in"=w346, "Image In"=w345, "Session In"=w344) -> ("error out"=w335:errorcluster, "Image Out"=w333:T3, "Session Out"=w338:T4)  [unwired: 5 in, 1 out]
    n98 = Wait (ms)(milliseconds to wait=u32 500) -> ()  [unwired: 1 out]
    n99 = call "IMAQ Copy"("error in (no error)"=w342, "Image Dst"=w341, "Image Src"=w333) -> ("error out"=w340:errorcluster, "Image Dst Out"=w339:T3)  [unwired: 3 in]
    n100 = call "SE FP Find red target.vi"("Image In"=w339, "error in (no error)"=w340) -> ("Image Dst Out"=w332:T3, "Nb Circles (Circle Detection 1)"=→"Nb Circles":i32, "Camera Data"=w331:T6, "error out"=w336:errorcluster)
    n101 = local write "Camera Data"(w331) -> ()
    n102 = local read "stop"() -> (w347:bool)
    n103 = Merge Errors(w335, w336) -> (w334:errorcluster)
  }
  n104 = while {
    shift-right: [w359] -> _
    shift-left: FALSE -> [w370]
    tunnel: w56 -> [w369]
    tunnel: [w363] -> w58
    stop <- w371 stop-if-true
    # "If myRIO battery is dead, STOP"
    # "Send command to \nthe hindbrain"
    # "Calculate the speed and heading\nusing an arbiter"
    # "Select Behaviors to use"
    # "Determine the status of the boat"
    # "Midbrain"
    n105 = local read "Boat Status"() -> (w354:T5)
    n106 = Wait (ms)(milliseconds to wait=u32 100) -> ()  [unwired: 1 out]
    n107 = Not(x=w370) -> (.not. x?=w359:bool)
    "Midbrain?" <- w359
    n108 = call "FP midbrain SENSE.vi"("Boat Status"=w354, "error in"=w369) -> ("IR Sensors"=w357:T8, "Battery\nDead?"=→"Battery Dead?":bool, "error out"=w367:errorcluster)
    n109 = local read "Forebrain Comd"() -> (w356:T10)
    n110 = shared-variable "CHRISTINE 2\\SVE variables.lvlib\\Tried Docking?"() -> (w351:bool)  [unwired: 1 in, 1 out]
    n111 = local read "Camera Data"() -> (w355:T6)
    n112 = local read "GPS Initial"() -> (w353:cluster{"X pos":i32, "Y pos":i32, "Heading":dbl})
    n113 = local read "GPS"() -> (w352:cluster{"X pos":i32, "Y pos":i32, "Heading":dbl})
    n114 = local read "TA GPS"() -> (w348:cluster{"X pos":i32, "Y pos":i32, "Heading":dbl})
    n115 = local read "In chase mode?"() -> (w349:bool)
    n116 = call "FP midbrain THINK.vi"("In chase mode?"=w349, "error in"=w367, "Camera Data"=w355, "IR Sensors"=w357, "GPS  Initial"=w353, "TA GPS"=w348, "Forebrain Comd"=w356, "GPS"=w352, "Tried Docking?"=w351) -> ("Behavior arrays"=w364:T36, "Behavior\nVelocity OUT"=w361:dbl, "Don't Use Forebrain ACT?"=w350:bool, "error out"=w366:errorcluster)  [unwired: 3 in]
    n117 = local read "Forebrain ACT"() -> (w362:dbl[])
    n118 = call "FP midbrain ACT.vi"("Forebrain ACT"=w362, "Behavior arrays"=w364, "Behavior\nVelocity"=w361, "error in"=w366, "Don't use Forebrain ACT?"=w350) -> ("Waveform Graph"=→"Arbiter Graph":cluster{dbl, dbl, dbl[]}, "Act Com"=w368:T7, "error out"=w363:errorcluster)
    n119 = local read "stop"() -> (w371:bool)
    n120 = local write "Act Com"(w368) -> ()
  }
  n121 = while {
    tunnel: w56 -> [w401]
    shift-right: [w389] -> _
    shift-left: FALSE -> [w390]
    tunnel: [w398] -> w54
    shift-right: [w394] -> _
    shift-left: w53 -> [w392]
    shift-right: [w380] -> _
    shift-left: w4 -> [w381]
    stop <- w402 stop-if-true
    # "Create a Command file and \nan arbiter array"
    # "Define the mission based upon the MDF"
    # "Get the boat status"
    # "Forebrain"
    n122 = local read "Boat Status"() -> (w396:T5)
    n123 = Not(x=w390) -> (.not. x?=w389:bool)
    "Forebrain?" <- w389
    n124 = shared-variable "CHRISTINE 2\\SVE variables.lvlib\\MDF"() -> (w374:T9)  [unwired: 1 in, 1 out]
    "MDF Active" <- w374
    n125 = Wait (ms)(milliseconds to wait=u32 500) -> ()  [unwired: 1 out]
    n126 = local read "MDF INDEX CHASE"() -> (w373:i32)
    n127 = call "FP forebrain SENSE.vi"("error in"=w401, "Boat Status"=w396) -> ("error out"=w400:errorcluster, "GPS"=w395:cluster{"X pos":i32, "Y pos":i32, "Heading":dbl})  [unwired: 1 in]
    n128 = shared-variable "CHRISTINE 2\\SVE variables.lvlib\\Tried Docking?"() -> (w384:bool)  [unwired: 1 in, 1 out]
    n129 = local read "Run?"() -> (w388:bool)
    n130 = local read "In chase mode?"() -> (w378:bool)
    n131 = local read "GPS Initial"() -> (w386:cluster{"X pos":i32, "Y pos":i32, "Heading":dbl})
    n132 = local read "GPS?"() -> (w379:bool)
    n133 = local read "Docking MDF"() -> (w382:T9)
    n134 = local read "Chase MDF"() -> (w375:T9)
    n135 = call "FP forebrain THINK.vi"("GPS"=w395, "MDF index"=w392, "GPS?"=w379, "MDF index docking"=w381, "Run?"=w388, "error in"=w400, "MDF in"=w374, "Tried Docking?"=w384, "MDF index chase"=w373, "Chase MDF In"=w375, "Docking MDF In"=w382, "In Chase Mode?"=w378, "GPS Initial"=w386) -> ("Docking MDF Out"=w383:T9, "Chase MDF Out"=w376:T9, "MDF Index out"=w394:i32, "Complete?"=→"Complete?":bool, "MDF Index out chase"=w372:i32, "Behaviors out"=w387:T37, "local Steering\nangle"=w393:dbl, "MDF Index out docking"=w380:i32, "Tried Docking? Output"=w385:bool, "In Chase Mode? Output"=w377:bool, "error out"=w399:errorcluster)  [unwired: 4 in]
    "MDF INDEX DOCKING" <- w380
    n136 = local write "Chase MDF"(w376) -> ()
    n137 = local write "Docking MDF"(w383) -> ()
    n138 = local write "In chase mode?"(w377) -> ()
    n139 = local write "Forebrain Comd"(w387) -> ()
    n140 = local write "MDF INDEX CHASE"(w372) -> ()
    n141 = call "FP forebrain ACT.vi"("error in"=w399, "local Steering\nangle"=w393, "Behaviors in"=w387) -> ("error out"=w398:errorcluster, "Forebrain ACT"=w397:dbl[])
    n142 = shared-variable "CHRISTINE 2\\SVE variables.lvlib\\Tried Docking?"(w385) -> ()  [unwired: 1 in, 1 out]
    n143 = local write "Forebrain ACT"(w397) -> ()
    n144 = local read "stop"() -> (w402:bool)
    "MDF INDEX" <- w392
  }
  n145 = call <vilib>:"IMAQdx Close Camera.vi"("error in"=w48, "Session In"=w47) -> ("error out"=w49:errorcluster)  [unwired: 9 out]
  n146 = call "IMAQ Dispose"("All Images? (No)"=TRUE, "Image"=w46, "error in (no error)"=w49) -> ("error out"=w45:errorcluster)  [unwired: 3 out]
  n147 = UDP Close(connection ID=w41, 8:w40) -> (error out=w39:errorcluster)  [unwired: 1 out]
  n148 = call <vilib>:"Close.vi"("error in (no error)"=w36, "AI Ref In"=w35) -> ("error out"=w17:errorcluster)  [unwired: 9 in]
  n149 = Build Array(w8, w8, w8, w8) -> (w11:bool[])
  n150 = call <vilib>:"Set Duty Cycle and Frequency.vi"("error in (no error)"=w28, "Frequency [Hz]"=w10, "Duty Cycle"=w9, "PWM Ref In"=w26) -> ("error out"=w27:errorcluster, "PWM Ref Out"=w25:T18)  [unwired: 5 in]
  n151 = call <vilib>:"Set Duty Cycle and Frequency.vi"("error in (no error)"=w24, "Frequency [Hz]"=w10, "Duty Cycle"=w9, "PWM Ref In"=w21) -> ("error out"=w23:errorcluster, "PWM Ref Out"=w22:T18)  [unwired: 5 in]
  n152 = call <vilib>:"Write.vi"("error in (no error)"=w15, "Values"=w11, "DIO Ref In"=w12) -> ("error out"=w14:errorcluster, "DIO Ref Out"=w13:T24)  [unwired: 6 in]
  n153 = call <vilib>:"Close.vi"("error in (no error)"=w14, "DIO Ref In"=w13) -> ("error out"=w18:errorcluster)  [unwired: 9 in]
  n154 = call <vilib>:"Close.vi"("error in (no error)"=w23, "PWM Ref In"=w22) -> ("error out"=w19:errorcluster)  [unwired: 9 in]
  n155 = call <vilib>:"Close.vi"("error in (no error)"=w27, "PWM Ref In"=w25) -> ("error out"=w20:errorcluster)  [unwired: 9 in]
  n156 = flat-sequence {
    tunnel: [w405] -> w7
    tunnel: w6 -> [w405]
    frame #0 {
      w404 = FALSE
      n157 = local write "Hindbrain?"(w404) -> ()
      n158 = local write "Complete?"(w404) -> ()
      n159 = local write "Midbrain?"(w404) -> ()
      n160 = local write "Forebrain?"(w404) -> ()
      n161 = local write "Complete?"(w404) -> ()
      n162 = local write "Manual?"(w404) -> ()
      n163 = local write "GLED"(w404) -> ()
      n164 = local write "RLED"(w404) -> ()
      n165 = local write "stop"(w404) -> ()
      n166 = local write "BLED"(w404) -> ()
      n167 = local write "Run?"(w404) -> ()
      n168 = local write "GPS?"(w404) -> ()
    }
  }
  n169 = Merge Errors(w17, w18, w19, w20) -> (w16:errorcluster)
  n170 = Merge Errors(w39, w45, w54, w58, w5, w16) -> (w6:errorcluster)
  "error out" <- w7
